vi "lvEtherbone.device_width.vi"(0 "eb_socket_ID":i32, 1 "eb_device_ID":i32, 5 "error in (no error)":errorcluster) -> (13 "eb_status":T2, 14 "eb_socket_ID out":i32, 15 "eb_device_ID out":i32, 16 "width":T1 items=["EB_DATA8"=1, "EB_DATA16"=2, "EB_DATA32"=4, "EB_DATA64"=8, "EB_DATAX"=15], 19 "error out":errorcluster)   [LabVIEW 2009, in "lvEtherbone.lvlib"]
doc: "//-----------------------------------------------------------------------------------\n// author : Dietrich Beck, GSI-Darmstadt\n// purpose : Recover the negotiated data width of the target device.\n// returns : lveb_status_t\n//-----------------------------------------------------------------------------------\nETHERBONE_API int lveb_device_width(int eb_deviceID, //ID of Wishbone device\n int *width //width of bus (eb_width_t)\n );"
uses:
  lvEtherbone.lvlib
  lvEtherbone.lveb_status_t.ctl
  lvEtherbone.eb_portWidth_t.ctl
  bin/lvEtherbone.dll
panel:
  in  "eb_width_t":T1 items=["EB_DATA8"=1, "EB_DATA16"=2, "EB_DATA32"=4, "EB_DATA64"=8, "EB_DATAX"=15]
  in  "myeb_status_t":T2
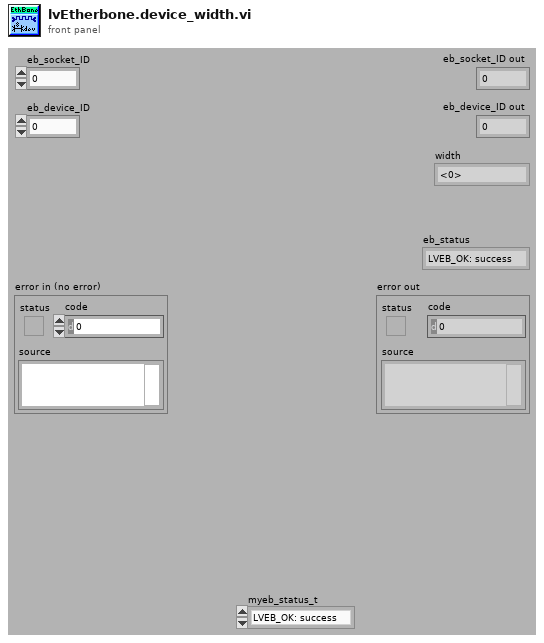
[diagram p1: front panel]
types:
  T1 = typedef "lvEtherbone.lvlib/lvEtherbone.eb_portWidth_t.ctl" = u32
  T2 = typedef "lvEtherbone.lvlib/lvEtherbone.lveb_status_t.ctl" = enum32{"LVEB_OK: success", "LVEB_UNKNOWN: unknown error", "LVEB_OS: operating system forbids access", "LVEB_PORT: port in use or unavailable", "LVEB_ID: ID invalid or out of resources", "LVEB_SOCKET: socket invalid or unavailable", "LVEB_EB: remote address is not Etherbone conformant", "LVEB_IP: bad format or network address", "LVEB_PORTWIDTH: port width error", "LVEB_DEVICEBUSY: Etherbone device still busy", "LVEB_DEVICEFAIL: operation on Wishbone device failed", "LVEB_DEVICEEXIST: Etherbone device already exists, overlaps, or does not exist", "LVEB_TIMEDOUT: a timeout occurred", "LVEB_OVERFLOW: payload of Etherbone exceeded", "LVEB_ADDRESS: bad address", "LVEB_ADDRESSWIDTH: address width error"}
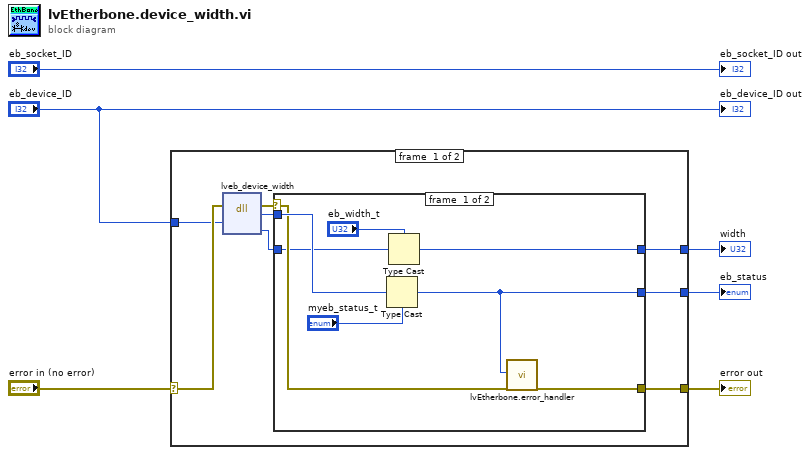
[diagram p0: block diagram]
diagram:
  n1 = case shown="No Error" "error in (no error)" {
    selector: "error in (no error)" -> [w14 w24]
    tunnel: [w7 w24] -> w5
    tunnel: "eb_device_ID" -> [w13 _]
    tunnel: [w9 _] -> w2
    tunnel: [w8 _] -> w1
    frame #0 {
      n2 = dll-call lib="F:/beck/Project/BEL/SCC/etherbone-core/api/lvEtherbone/bin/lvEtherbone.*" fn="lveb_device_width"(error in=w14, "eb_device_ID"=w13) -> (error out=w12:errorcluster, "myeb_status_t"=w11:i32, "width"=w10:i32)  [unwired: 4 in, 1 out]
      n3 = case shown="No Error" w12 {
        selector: w12 -> [w19 w23]
        tunnel: w11 -> [w22 _]
        tunnel: [w18 _] -> w9
        tunnel: [w20 w23] -> w7
        tunnel: w10 -> [w17 _]
        tunnel: [w15 _] -> w8
        frame #0 {
          n4 = Type Cast(type="myeb_status_t", x=w22) -> (*(type *) &x=w18:T2)
          n5 = Type Cast(type="eb_width_t", x=w17) -> (*(type *) &x=w15:T1)
          n6 = call "lvEtherbone.error_handler.vi"("eb_status"=w18, "error in"=w19) -> ("error out"=w20:errorcluster)  [unwired: 17 in]
        }
        frame #1 {
        }
      }
    }
    frame #1 {
    }
  }
  "error out" <- w5
  "width" <- w1
  "eb_status" <- w2
  "eb_socket_ID out" <- "eb_socket_ID"
  "eb_device_ID out" <- "eb_device_ID"
